vi "Get ECU Name.vi"(8 "Type (Input)":T3, 9 "ECUs":T4[](array[typedef]), 10 "Frame":T1, 11 "Frames":T1[](array[typedef])) -> (2 "Found?":bool, 3 "ECU Name":string)   [LabVIEW 2020, in "Communication Bus Template System Explorer.lvlib" / "Implementation.lvlib"]
uses:
  Implementation.lvlib
  Types/ECU.ctl
  <vilib>/NI VeriStand/Custom Device API/Custom Device Channel Type.ctl
  Types/Frame.ctl
  Types/Signal.ctl
  <vilib>/NI VeriStand/Custom Device API/Custom Device API.lvlib
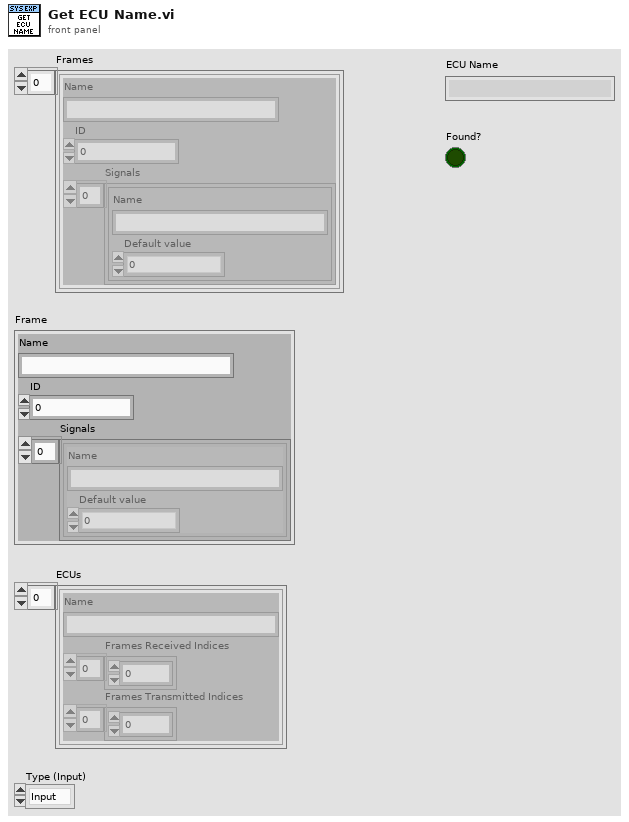
[diagram p1: front panel]
types:
  T1 = typedef "Communication Bus Template System Explorer.lvlib/Implementation.lvlib/Frame.ctl" = cluster{"Name":string, "ID":u32, "Signals":T2[]}
  T2 = typedef "Communication Bus Template System Explorer.lvlib/Implementation.lvlib/Signal.ctl" = cluster{"Name":string, "Default value":dbl}
  T3 = typedef "Custom Device API.lvlib/Custom Device Channel Type.ctl" = enum16{"Input", "Output"}
  T4 = typedef "Communication Bus Template System Explorer.lvlib/Implementation.lvlib/ECU.ctl" = cluster{"Name":string, "Frames Received Indices":u32[], "Frames Transmitted Indices":u32[]}
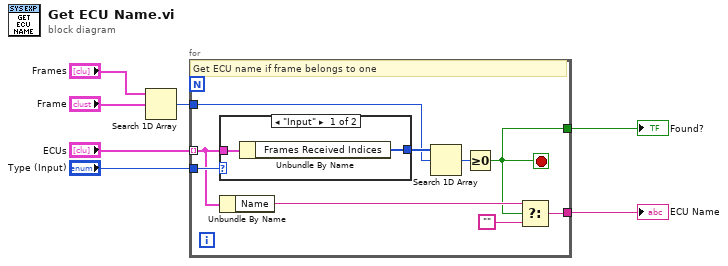
[diagram p0: block diagram]
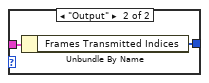
[diagram p2: hidden frame]
diagram:
  n1 = Search 1D Array(1D array="Frames", element="Frame") -> (index of element=w7:i32)  [unwired: 1 in]
  n2 = for {
    tunnel: w7 -> [w13]
    tunnel: "ECUs" -> [w15] mode=indexing
    tunnel: "Type (Input)" -> [w16]
    tunnel: [w9] -> w2
    tunnel: [w8] -> w1
    stop <- w8 stop-if-true
    # "Get ECU name if frame belongs to one"
    n3 = case shown="\"Input\"" w16 {
      tunnel: w15 -> [w18 w20]
      tunnel: [w17 w19] -> w14
      frame "Input" {
        n4 = Unbundle By Name(w18) -> ("Frames Received Indices"=w17:u32[])
      }
      frame "Output" {
        n5 = Unbundle By Name(w20) -> ("Frames Transmitted Indices"=w19:u32[])
      }
    }
    n6 = Unbundle By Name(w15) -> ("Name"=w11:string)
    n7 = Search 1D Array(1D array=w14, element=w13) -> (index of element=w12:i32)  [unwired: 1 in]
    n8 = Greater Or Equal To 0?(x=w12) -> (x >= 0?=w8:bool)
    n9 = Select(t=w11, s=w8, f="") -> (s? t:f=w9:string)
  }
  "ECU Name" <- w2
  "Found?" <- w1
